vi "get sync in settings.vi"(8 "error in (no error)":errorcluster, 10 "sync_in_settings":T1, 11 "id":i32) -> (0 "error out":errorcluster, 2 "sync_in_settings out":T1, 3 "function return":i32)   [LabVIEW 2012, in "libximc.lvlib"]
doc: "result_t XIMC_API get_sync_in_settings (device_t id, sync_in_settings_t* sync_in_settings);"
uses:
  libximc.lvlib
  libximc.dll
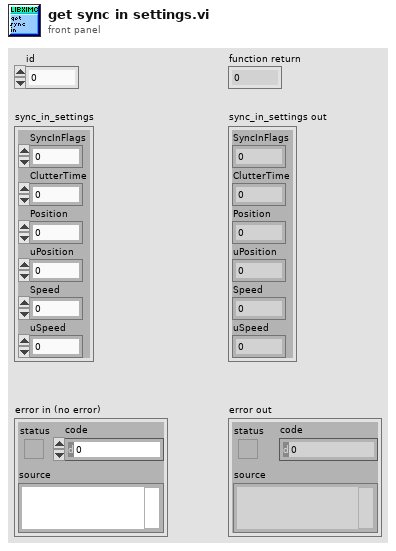
[diagram p1: front panel]
types:
  T1 = cluster{"SyncInFlags":u32, "ClutterTime":u32, "Position":i32, "uPosition":i32, "Speed":u32, "uSpeed":u32}
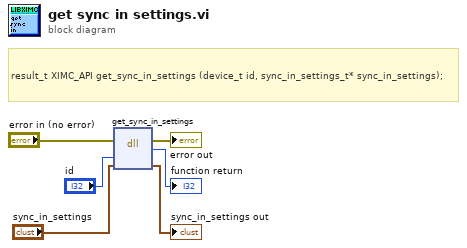
[diagram p0: block diagram]
diagram:
  # "result_t XIMC_API get_sync_in_settings (device_t id, sync_in_settings_t* sync_in_settings);"
  n1 = dll-call lib="C:/Users/user/Desktop/labview-2.9.11-gen/libximc.*" fn="get_sync_in_settings"(error in="error in (no error)", "id"="id", "sync_in_settings"="sync_in_settings") -> (error out=→"error out":errorcluster, →"function return":i32, "sync_in_settings"=→"sync_in_settings out":T1)  [unwired: 3 in, 1 out]
